vi "util_transparency.vi"(7 "vi_reference":refnum<vi>, 8 "error in (no error)":errorcluster, 10 "wait_ms":u32=25, 11 "opaque_transparent":bool) -> (0 "error out":errorcluster)   [LabVIEW 2015, in "lv-launcher-nre.lvlib"]
uses:
  lv-launcher-nre.lvlib
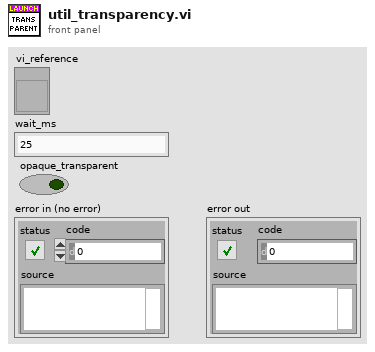
[diagram p1: front panel]
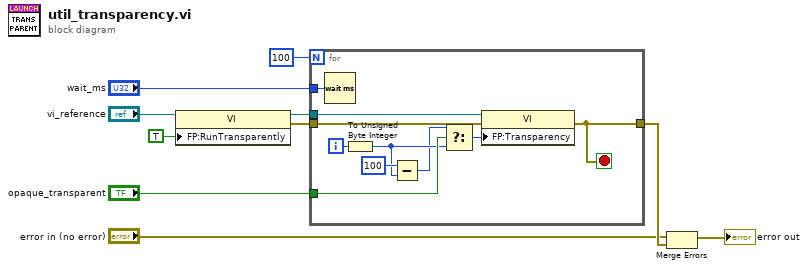
[diagram p0: block diagram]
diagram:
  n1 = property class="VI"(reference="vi_reference", "FP:RunTransparently"=TRUE ("Front Panel Window:Run VI Transparently")) -> (reference out=w4:refnum<vi>, error out=w3:errorcluster)  [unwired: 1 in]
  n2 = for {
    N: 100 -> [_]
    tunnel: w4 -> [w20]
    tunnel: "wait_ms" -> [w16]
    tunnel: "opaque_transparent" -> [w14]
    tunnel: w3 -> [w19]
    tunnel: [w17] -> w7
    i -> [w18]
    stop <- w17 stop-if-true
    n3 = Wait (ms)(milliseconds to wait=w16) -> ()  [unwired: 1 out]
    n4 = To Unsigned Byte Integer(number=w18) -> (unsigned 8bit integer=w13:u8)
    n5 = Subtract(x=u8 100, y=w13) -> (x-y=w12:u8)
    n6 = Select(t=w12, s=w14, f=w13) -> (s? t:f=w11:u8)
    n7 = property class="VI"(reference=w20, error in=w19, "FP:Transparency"=w11) -> (error out=w17:errorcluster)  [unwired: 1 out]
  }
  n8 = Merge Errors("error in (no error)", w7) -> (→"error out":errorcluster)
